vi "Begin.vi"(8 "error in":errorcluster) -> (0 "error out":errorcluster)   [LabVIEW 2023]
doc: "Called before other user functions, this VI is expected to open initial I/O refnums, load in file data, and do all program initialization. Notice that the <B>error out</B> terminal is simply used for data flow. Wiring it to other structures or subVIs ensures that this VI runs first."
uses:
  <vilib>/Rock Robotics/Network Tables/NT Write String Array.vi
  RoboRIO Utilities/Global_STOP.vi
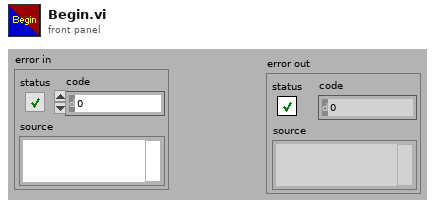
[diagram p1: front panel]
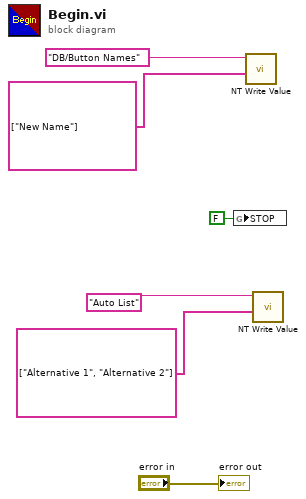
[diagram p0: block diagram]
diagram:
  n1 = global write "Global_STOP.vi" "STOP"(FALSE ("STOP")) -> ()
  n2 = call-poly <vilib>:"NT Write Value.vi"("value"=string[] ["New Name"], "name"="DB/Button Names" ("Name")) -> ()  [unwired: 9 in, 1 out]
  n3 = call-poly <vilib>:"NT Write Value.vi"("value"=string[] ["Alternative 1", "Alternative 2"] ("String Array"), "name"="Auto List" ("Name")) -> ()  [unwired: 9 in, 1 out]
  "error out" <- "error in"
